vi "text decryption.vi"() -> ()   [LabVIEW 2022 SP3]
uses:
  <vilib>/Analysis/2dsp.llb/Inverse Real FFT.vi
  <vilib>/Analysis/NI_AALPro.lvlib
panel:
  in  "Error in":errorcluster
  out "Result string":string
  out "Output data":cdb[](array[numeric])
  out "Data":cdb[](array[numeric])
  in  "Array":cdb[](array[numeric])
  in  "Read/write":enum16{"read/write", "read-only", "write-only"}(ring)
  in  "Open":T1(ring)
  in  "File path":path
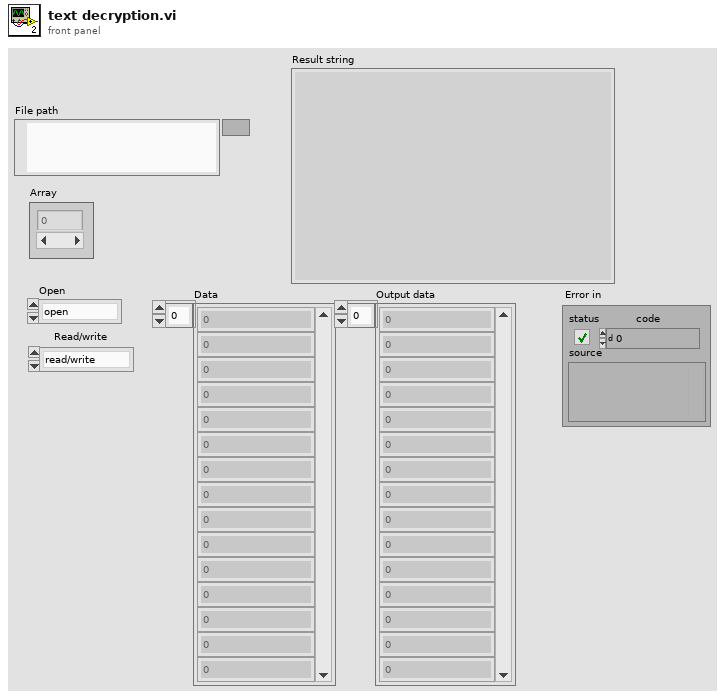
[diagram p1: front panel]
types:
  T1 = enum16{"open", "replace", "create", "open or create", "replace or create", "replace or create with confirmation"}
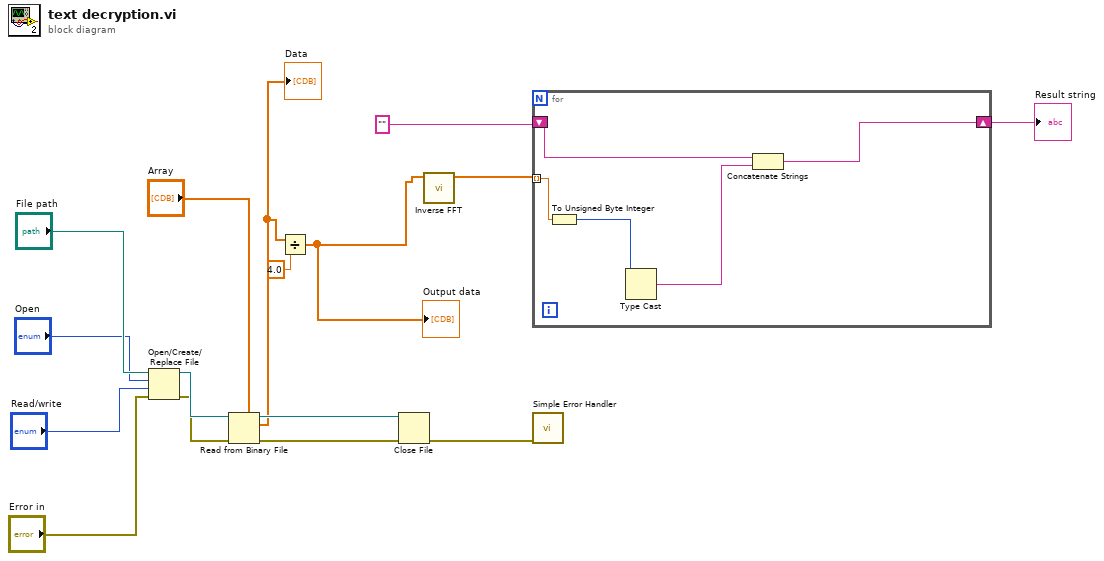
[diagram p0: block diagram]
diagram:
  n1 = Open/Create/Replace File(file path (use dialog)="File path", error in="Error in", operation (0:open)="Open", access (0:read/write)="Read/write") -> (refnum out=w13:refnum<file>, error out=w11:errorcluster)  [unwired: 2 in, 1 out]
  n2 = Read from Binary File(5:"Array", 8:w11, 11:w13) -> (0:w10:errorcluster, 2:w7:cdb[], 3:w12:refnum<file>)  [unwired: 3 in, 1 out]
  "Data" <- w7
  n3 = Divide(x=w7, y=4.0) -> (x/y=w6:cdb[])
  "Output data" <- w6
  n4 = Close File(refnum=w12, error in=w10) -> (error out=w9:errorcluster)  [unwired: 1 out]
  n5 = call-poly <vilib>:"Inverse FFT.vi"("FFT {X}"=w6) -> ("X"=w5:dbl[])  [unwired: 9 in, 1 out]
  n6 = for {
    tunnel: w5 -> [w21] mode=indexing
    shift-right: [w17] -> w1
    shift-left: "" -> [w18]
    n7 = To Unsigned Byte Integer(number=w21) -> (unsigned 8bit integer=w20:u8)
    n8 = Type Cast(x=w20) -> (*(type *) &x=w19:string)  [unwired: 1 in]
    n9 = Concatenate Strings "Concatenate Strings"(w18, w19) -> (w17:string)
  }
  "Result string" <- w1
  n10 = call <vilib>:"Simple Error Handler.vi"("error in (no error)"=w9) -> ()  [unwired: 4 in, 5 out]
